vi "AcquireCalculateDroppedFrames.vi"(9 "LastBuffer":u32, 10 "CurrentBuffer":u32, 11 "DroppedFrames":u32) -> (2 "CurrentBufferOut":u32, 3 "DroppedOut":u32)   [LabVIEW 2017, in "ImageAcquisitionLibrary.lvlib"]
uses:
  ImageAcquisitionLibrary.lvlib
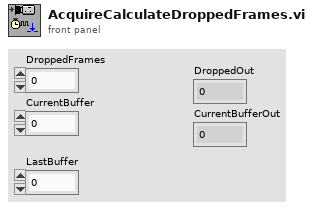
[diagram p1: front panel]
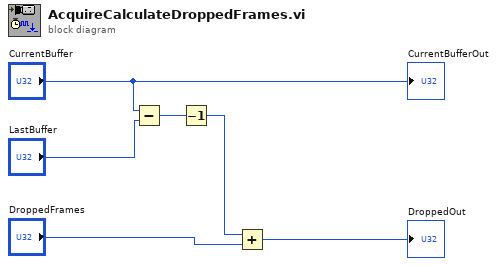
[diagram p0: block diagram]
diagram:
  n1 = Subtract(x="CurrentBuffer", y="LastBuffer") -> (x-y=w5:u32)
  n2 = Decrement(x=w5) -> (x-1=w3:u32)
  n3 = Add(x=w3, y="DroppedFrames") -> (x+y=→"DroppedOut":u32)
  "CurrentBufferOut" <- "CurrentBuffer"
